vi "testKM.vi"() -> ()   [LabVIEW 2014]
panel:
  in  "count 2":dbl
  in  "count":dbl
  in  "R":dbl
  in  "s":dbl
  out "Frequency 2":dbl
  in  "Frequency":dbl=10.1
  in  "Amplitude":dbl=1.0
  out "Sine":dynamicdata(graph)
  in  "stop":bool
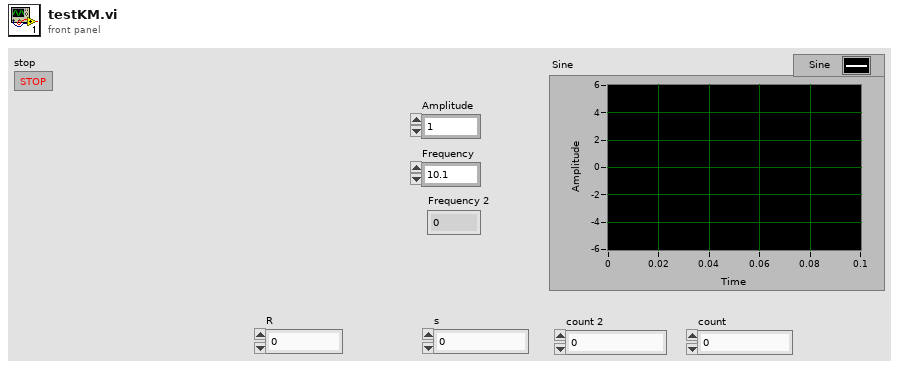
[diagram p1: front panel]
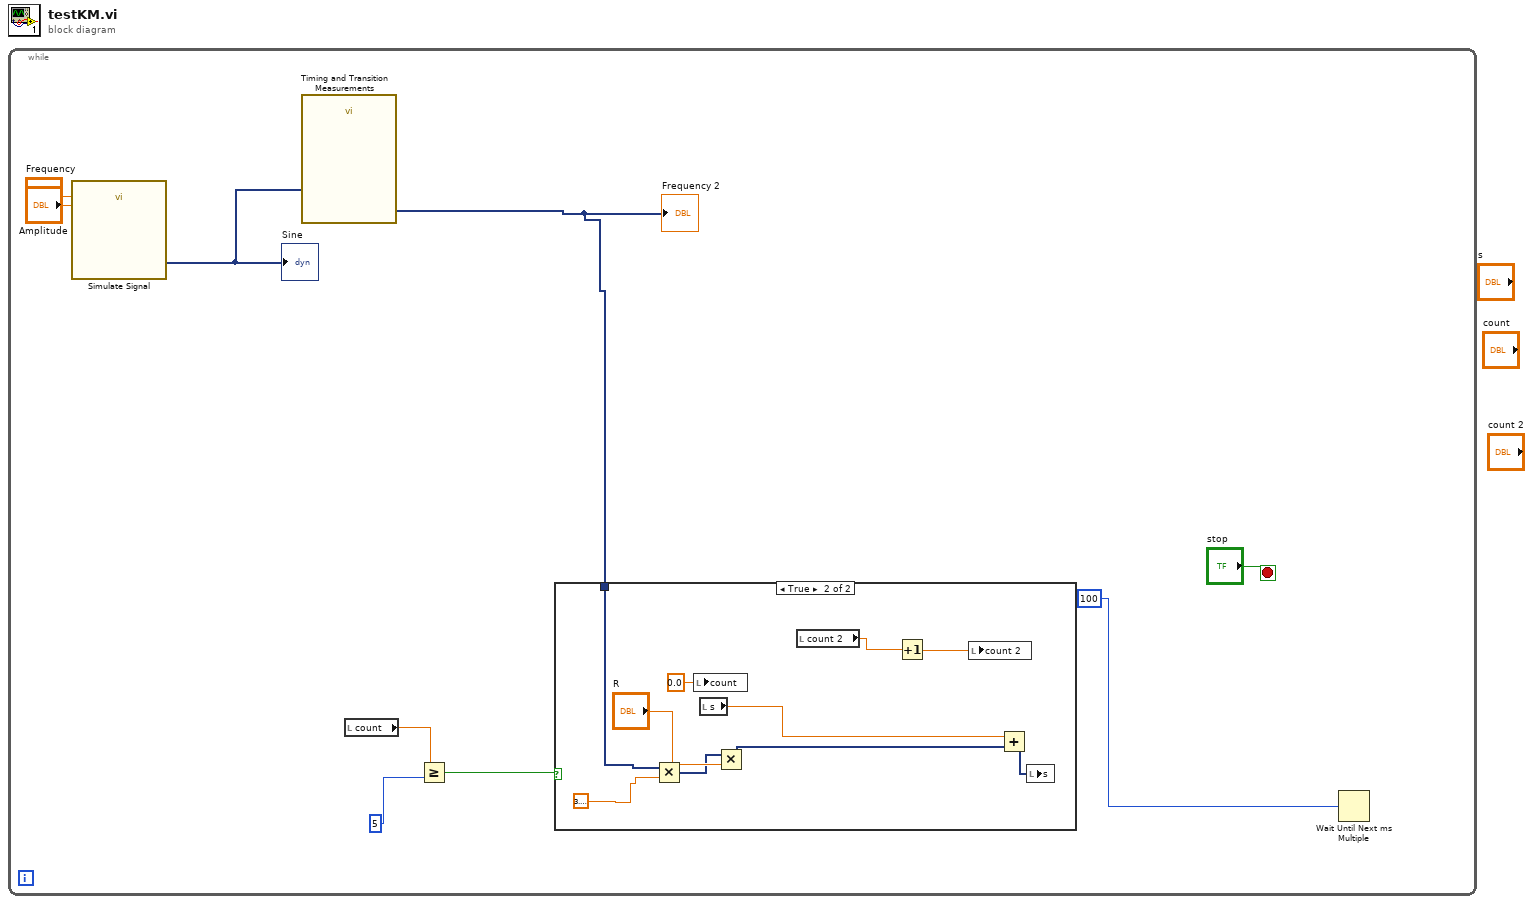
[diagram p0: block diagram]
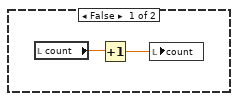
[diagram p2: hidden frame]
diagram:
  n1 = while {
    stop <- "stop" stop-if-true
    n2 = call "Simulate Signal"("Frequency"="Frequency", "Amplitude"="Amplitude") -> ("Sine"=w7:dynamicdata)  [unwired: 12 in, 1 out]
    "Sine" <- w7
    n3 = call "Timing and Transition Measurements"("Signals"=w7) -> ("Frequency"=w1:dynamicdata)  [unwired: 9 in, 1 out]
    "Frequency 2" <- w1
    n4 = local read "count"() -> (w5:dbl)
    n5 = Greater Or Equal?(x=w5, y=5) -> (x >= y?=w3:bool)
    n6 = case shown="True" w3 {
      tunnel: w1 -> [_ w19]
      frame False {
        n7 = local read "count"() -> (w11:dbl)
        n8 = Increment(x=w11) -> (x+1=w10:dbl)
        n9 = local write "count"(w10) -> ()
      }
      frame True {
        n10 = Multiply(x=w19, y=3.141592653589793) -> (x*y=w20:dynamicdata)
        n11 = local write "count"(0.0 ("count")) -> ()
        n12 = local read "s"() -> (w16:dbl)
        n13 = Multiply(x=w20, y="R") -> (x*y=w17:dynamicdata)
        n14 = local read "count 2"() -> (w13:dbl)
        n15 = Increment(x=w13) -> (x+1=w12:dbl)
        n16 = local write "count 2"(w12) -> ()
        n17 = Add(x=w16, y=w17) -> (x+y=w15:dynamicdata)
        n18 = local write "s"(w15) -> ()
      }
    }
    n19 = Wait Until Next ms Multiple(millisecond multiple=u32 100) -> ()  [unwired: 1 out]
  }
